vi "LINETEST.vi"   [LabVIEW 2019]
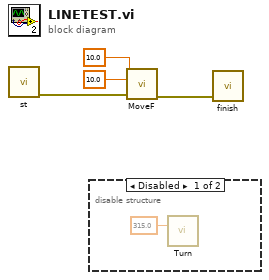
[diagram p0: block diagram]
diagram:
  n1 = call "st.vi"() -> ("Error/Flow Out"=w2:errorcluster)  [unwired: 11 in]
  n2 = disable-structure shown="Disabled" {
    frame Disabled {
      n3 = call "Turn.vi"("¨¤«×"=315.0) -> ()  [unwired: 14 in, 1 out]
    }
    frame Enabled {
    }
  }
  n4 = call "MoveF.vi"("X"=10.0, "Y"=10.0, "error in (no error)"=w2) -> ("error out"=w1:errorcluster)  [unwired: 12 in]
  n5 = call "finish.vi"("Error/Flow In"=w1) -> ()  [unwired: 11 in]
